vi "Autonomous Independent.vi"() -> ()   [LabVIEW 2016]
doc: "This VI is called when autonomous begins, and will automatically be terminated when autonomous ends. You can carry out timed or sensor driven robot movement independently without needing to return to the caller."
uses:
  <vilib>/Rock Robotics/Network Tables/NT Read Number.vi
  1_25_17/Action_type_def.ctl
  <vilib>/Rock Robotics/WPI/Solenoid/WPI_SolenoidValue.ctl
panel:
  in  "Value":T1=enum."Forward"
  out "Defense Type":dbl=3.0
  in  "Auton_Modes":T3(array[cluster])=[{"Actions"=[{"Action"=enum."Drive", "Effort"=0.55, "Duration"=3.5}, {"Action"=enum."Nothing", "Effort"=0.0, "Duration"=0.0}]}, {"Actions"=[{"Action"=enum."Art Down", "Effort"=0.0, "Duration"=1.0}, {"Action"=enum."Drive", "Effort"=0.75, "Duration"=5.0}, {"Action"=enum."Art Up", "Effort"=0.0, "Duration"=1.0}]}, {"Actions"=[{"Action"=enum."Drive", "Effort"=1.0, "Duration"=3.0}, {"Action"=enum."Art Down", "Effort"=0.0, "Duration"=1.0}, {"Action"=enum."Drive", "Effort"=0.75, "Duration"=3.5}, {"Action"=enum."Art Up", "Effort"=0.0, "Duration"=1.0}]}, {"Actions"=[{"Action"=enum."Art Down", "Effort"=0.0, "Duration"=0.5}, {"Action"=enum."Drive", "Effort"=0.8, "Duration"=5.28}, {"Action"=enum."Art Up", "Effort"=0.0, "Duration"=1.0}, {"Action"=enum."Turn", "Effort"=-0.8, "Duration"=1.8}, {"Action"=enum."Nothing", "Effort"=0.0, "Duration"=0.1}, {"Action"=enum."Drive", "Effort"=0.8, "Duration"=1.75}, {"Action"=enum."Art Down", "Effort"=0.0, "Duration"=0.5}, {"Action"=enum."climb", "Effort"=0.0, "Duration"=4.0}]}, {"Actions"=[{"Action"=enum."Shift", "Effort"=0.0, "Duration"=0.0}, {"Action"=enum."Drive", "Effort"=1.0, "Duration"=0.1}, {"Action"=enum."Nothing", "Effort"=0.0, "Duration"=0.1}, {"Action"=enum."Drive", "Effort"=1.0, "Duration"=3.0}]}, {"Actions"=[{"Action"=enum."Shift", "Effort"=0.0, "Duration"=0.0}, {"Action"=enum."Drive", "Effort"=1.0, "Duration"=0.1}, {"Action"=enum."Nothing", "Effort"=0.0, "Duration"=0.1}, {"Action"=enum."Drive", "Effort"=1.0, "Duration"=3.0}]}, {"Actions"=[{"Action"=enum."Drive", "Effort"=0.55, "Duration"=4.0}, {"Action"=enum."Art Down", "Effort"=0.0, "Duration"=1.0}, {"Action"=enum."Drive", "Effort"=-0.5, "Duration"=0.6}, {"Action"=enum."Drive", "Effort"=0.75, "Duration"=1.0}, {"Action"=enum."Art Up", "Effort"=0.0, "Duration"=1.0}, {"Action"=enum."Drive", "Effort"=0.75, "Duration"=3.0}]}, {"Actions"=[{"Action"=enum."Art Down", "Effort"=0.0, "Duration"=0.5}, {"Action"=enum."Drive", "Effort"=0.55, "Duration"=4.25}, {"Action"=enum."Art Up", "Effort"=0.0, "Duration"=0.0}, {"Action"=enum."Nothing", "Effort"=0.0, "Duration"=0.3}, {"Action"=enum."Drive", "Effort"=0.9, "Duration"=2.0}]}, {"Actions"=[{"Action"=enum."Nothing", "Effort"=0.0, "Duration"=0.0}]}]
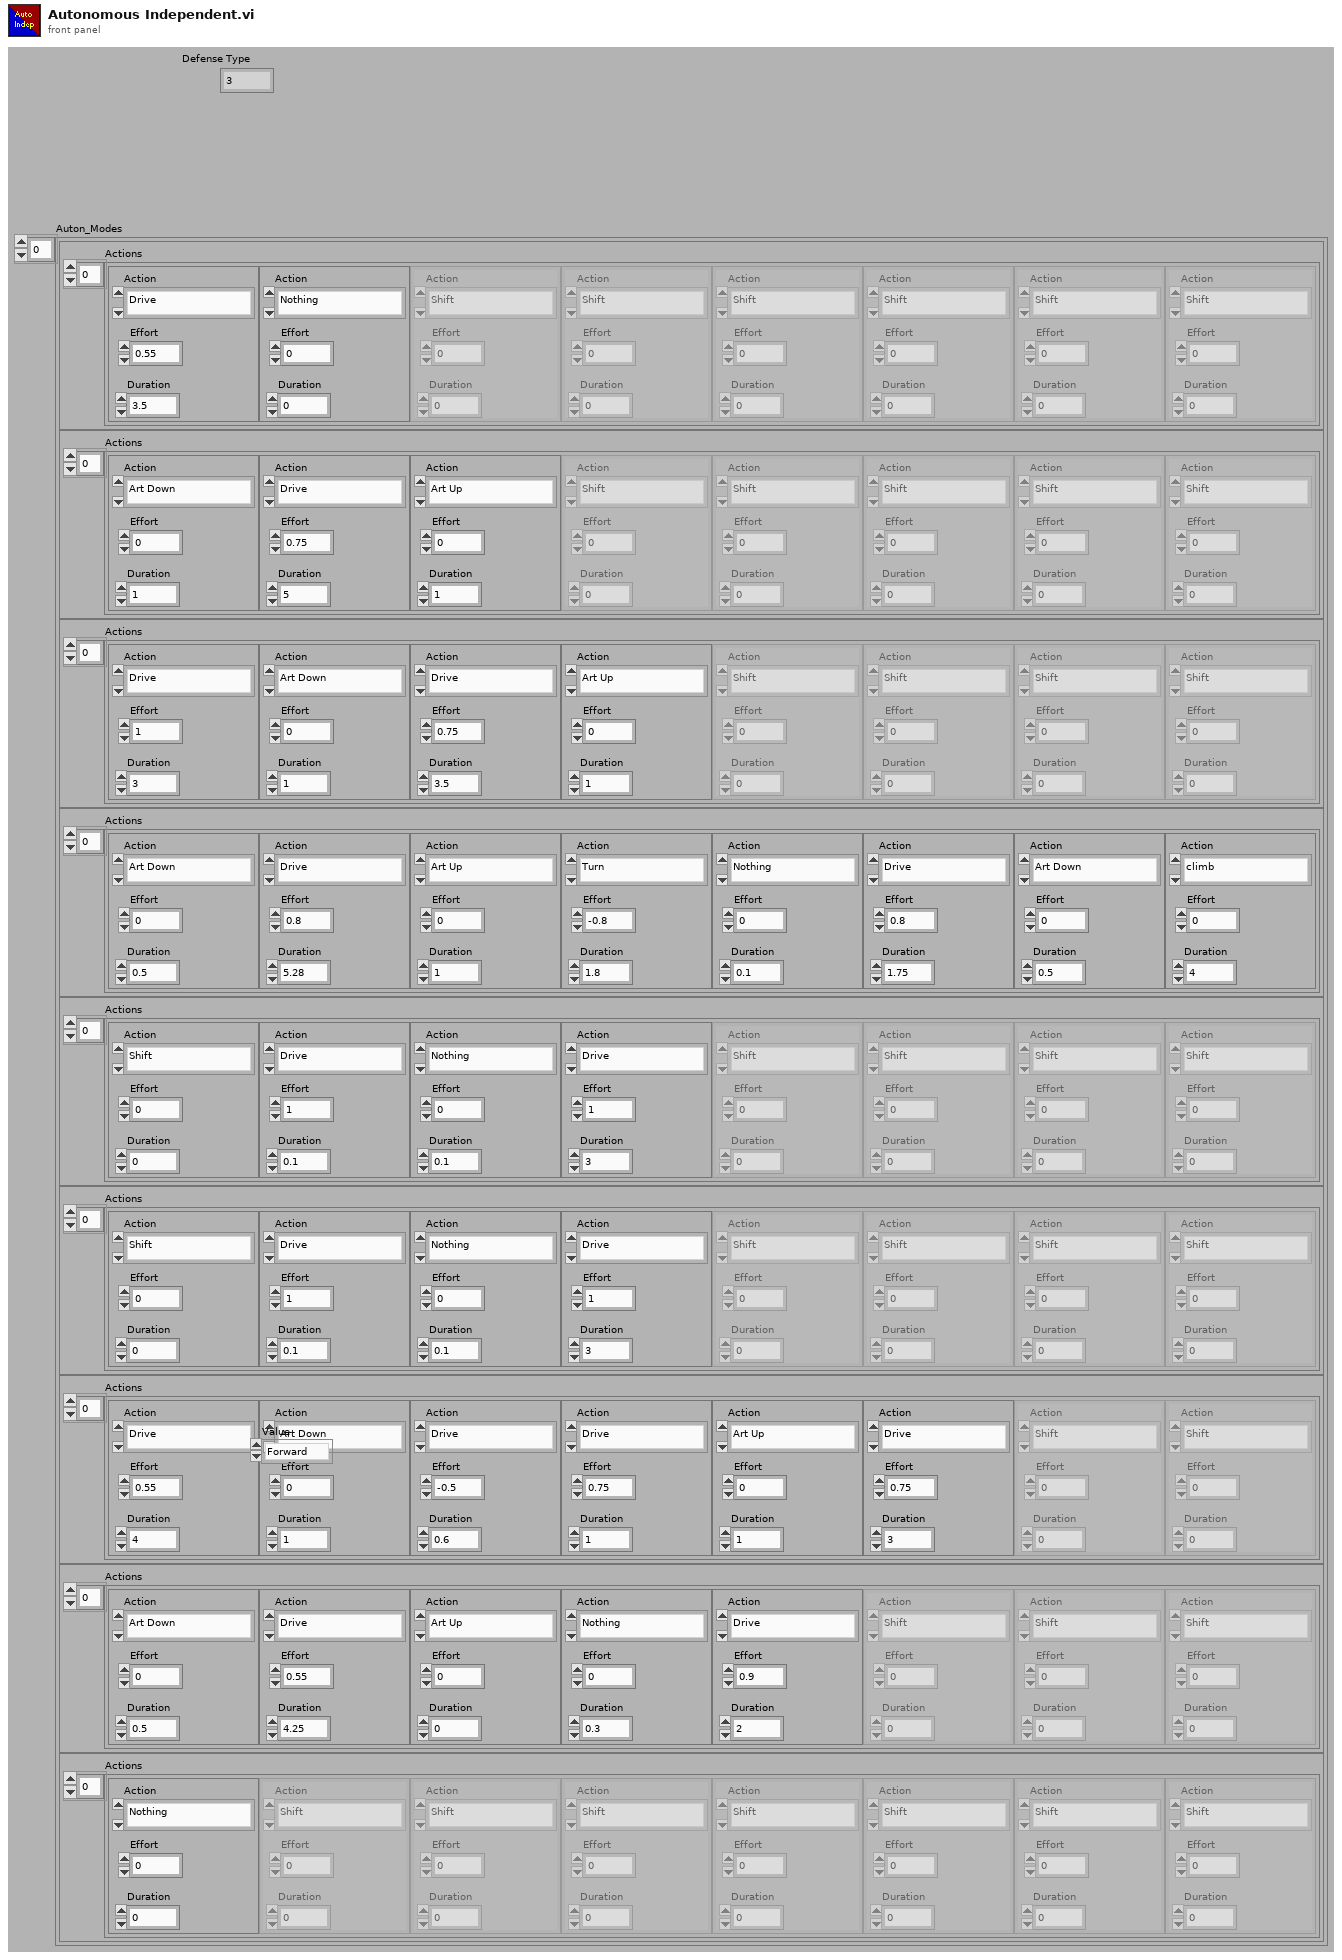
[diagram p1: front panel]
types:
  T1 = typedef "WPI_SolenoidValue.ctl" = enum16{"Off", "On", "Forward", "Reverse"}
  T2 = typedef "Action_type_def.ctl" = enum16{"Shift", "Shoot", "Move Articulates", "Nothing", "Drive", "Turn", "climb", "Art Up", "Art Down", "Test"}
  T3 = cluster{"Actions":cluster{"Action":T2, "Effort":dbl, "Duration":dbl}[]}[]
  T4 = cluster{"Actions":cluster{"Action":T2, "Effort":dbl, "Duration":dbl}[]}
  T5 = cluster{"Action":T2, "Effort":dbl, "Duration":dbl}[]
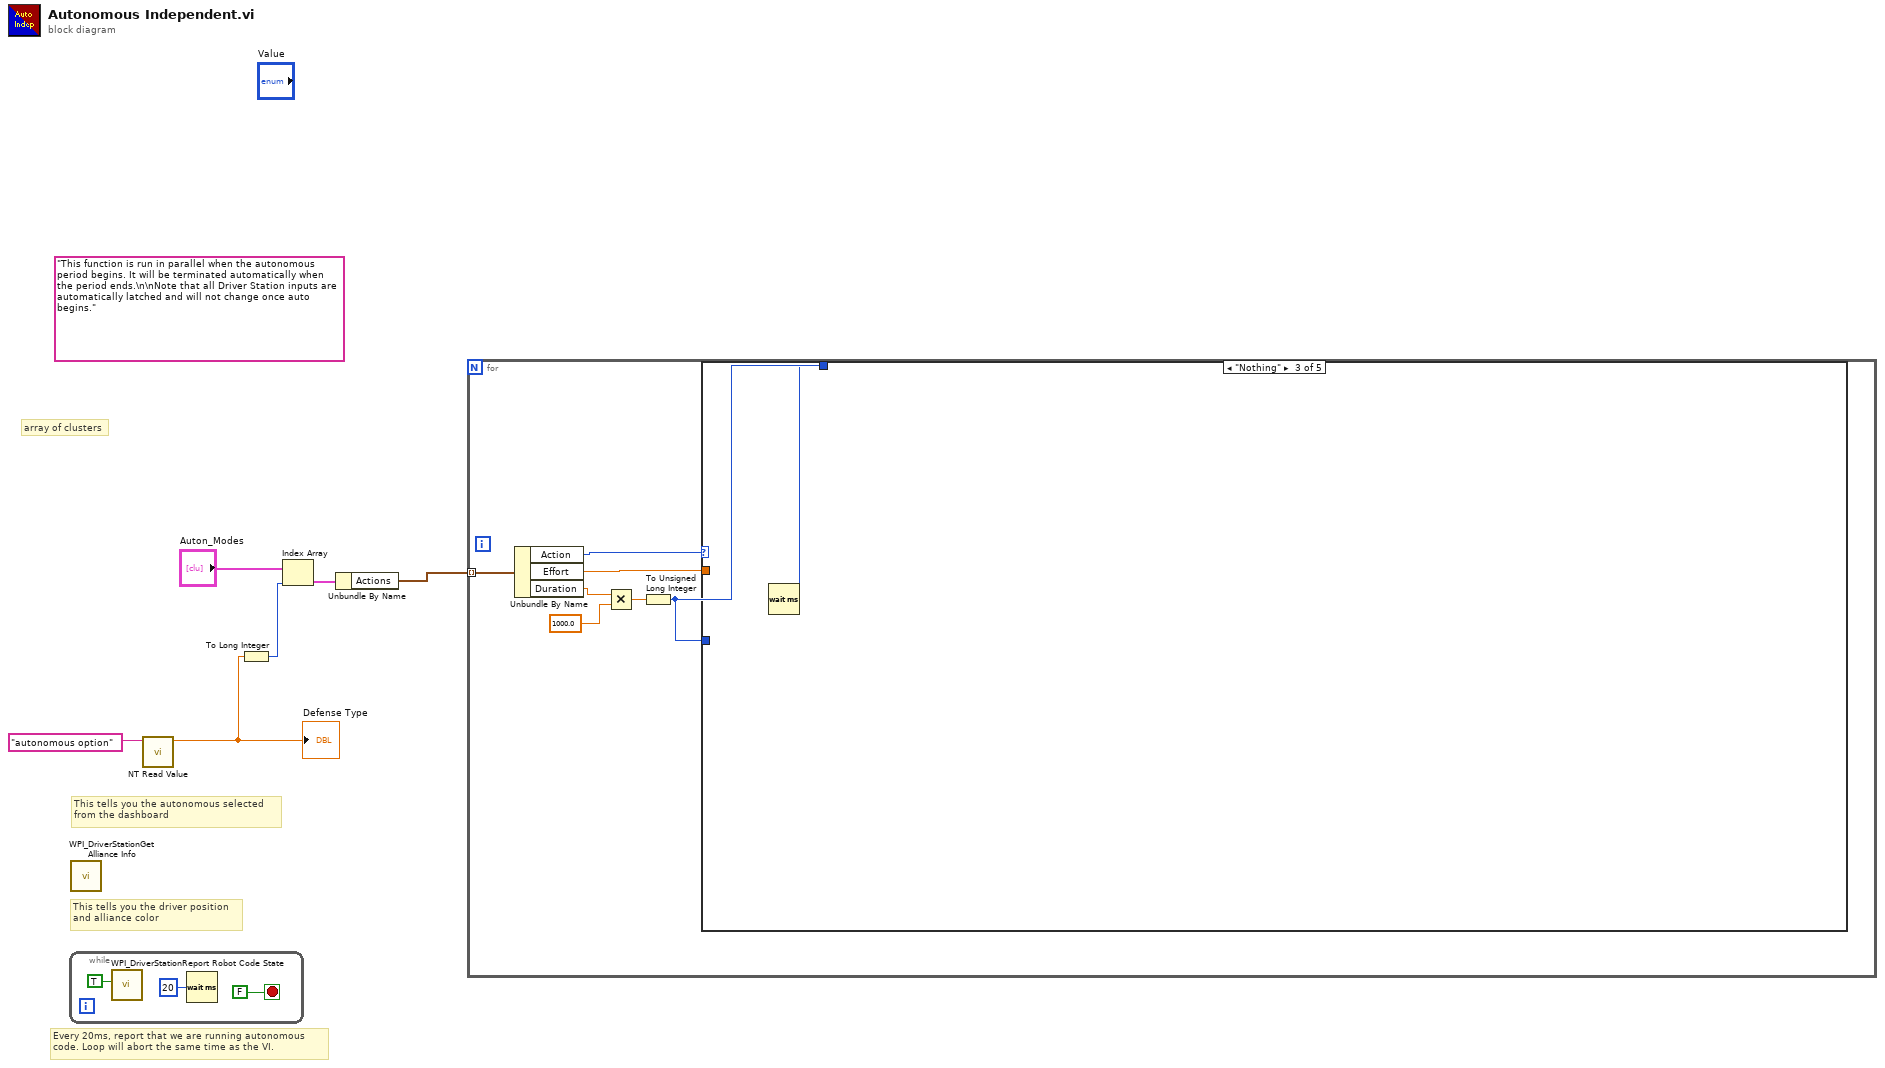
[diagram p0: block diagram]
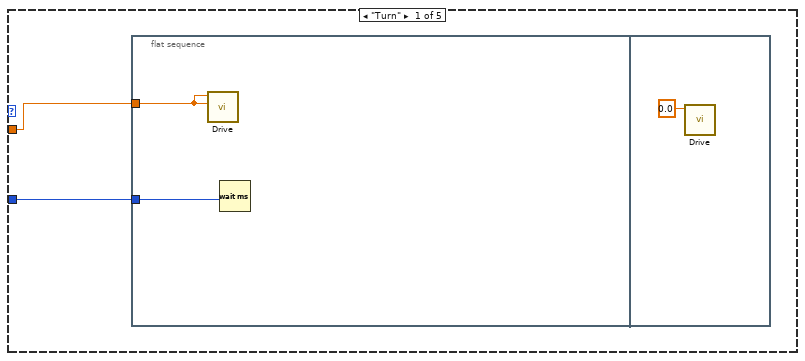
[diagram p2: hidden frame]
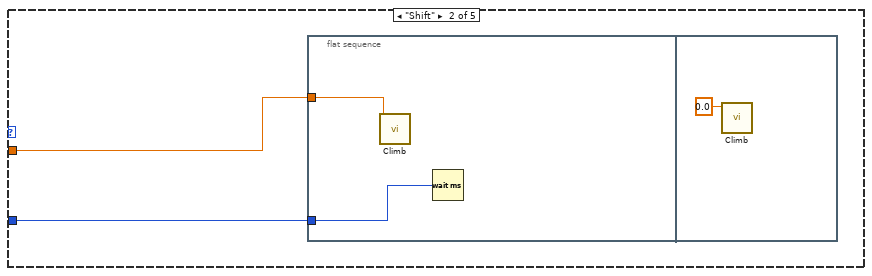
[diagram p3: hidden frame]
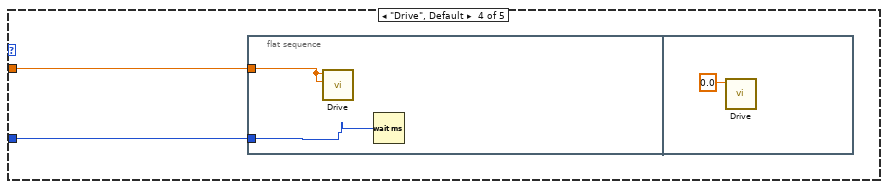
[diagram p4: hidden frame]
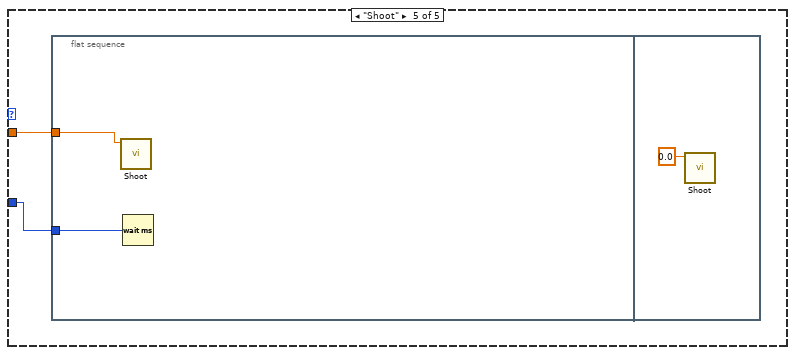
[diagram p5: hidden frame]
diagram:
  (unwired) "This function is run in parallel when the autonomous period begins. It will be terminated automatically when the period ends.\n\nNote that all Driver Station inputs are automatically latched and will not change once auto begins."
  # "This tells you the autonomous selected\nfrom the dashboard"
  # "array of clusters"
  # "Every 20ms, report that we are running autonomous\ncode. Loop will abort the same time as the VI."
  # "This tells you the driver position\nand alliance color"
  n1 = while {
    stop <- FALSE stop-if-true
    n2 = call <vilib>:"WPI_DriverStationReport Robot Code State.vi"("Autonomous"=TRUE) -> ()  [unwired: 10 in, 1 out]
    n3 = Wait (ms)(milliseconds to wait=u32 20) -> ()  [unwired: 1 out]
  }
  n4 = call <vilib>:"WPI_DriverStationGet Alliance Info.vi"() -> ()  [unwired: 12 out]
  n5 = call-poly <vilib>:"NT Read Value.vi"("Name"="autonomous option") -> ("Numeric"=w1:dbl)  [unwired: 9 in, 1 out]
  "Defense Type" <- w1
  n6 = To Long Integer(number=w1) -> (32bit integer=w3:i32)
  n7 = Index Array(array="Auton_Modes", index=w3) -> (element=w5:T4)
  n8 = Unbundle By Name(w5) -> ("Actions"=w6:T5)
  n9 = for {
    tunnel: w6 -> [w16] mode=indexing
    n10 = Unbundle By Name(w16) -> ("Action"=w15:T2, "Effort"=w14:dbl, "Duration"=w13:dbl)
    n11 = Multiply(x=w13, y=1000.0) -> (x*y=w11:dbl)
    n12 = To Unsigned Long Integer(number=w11) -> (unsigned 32bit integer=w10:u32)
    n13 = case shown="\"Nothing\"" w15 {
      tunnel: w14 -> [w18 w23 _ w29 w34]
      tunnel: w10 -> [_ _ w27 _ _]
      tunnel: w10 -> [w17 w22 _ w28 w33]
      frame "Turn" {
        n14 = flat-sequence {
          tunnel: w18 -> [w20]
          tunnel: w17 -> [w19]
          frame #0 {
            n15 = call "Drive.vi"("Drive R"=w20, "Drive L"=w20) -> ()  [unwired: 10 in]
            n16 = Wait (ms)(milliseconds to wait=w19) -> ()  [unwired: 1 out]
          }
          frame #1 {
            n17 = call "Drive.vi"("Drive L"=0.0) -> ()  [unwired: 11 in]
          }
        }
      }
      frame "Shift" {
        n18 = flat-sequence {
          tunnel: w23 -> [w25]
          tunnel: w22 -> [w24]
          frame #0 {
            n19 = call "Climb.vi"("Effort"=w25) -> ()  [unwired: 11 in]
            n20 = Wait (ms)(milliseconds to wait=w24) -> ()  [unwired: 1 out]
          }
          frame #1 {
            n21 = call "Climb.vi"("Effort"=0.0) -> ()  [unwired: 11 in]
          }
        }
      }
      frame "Nothing" {
        n22 = Wait (ms)(milliseconds to wait=w27) -> ()  [unwired: 1 out]
      }
      frame "Drive", Default {
        n23 = flat-sequence {
          tunnel: w29 -> [w31]
          tunnel: w28 -> [w30]
          frame #0 {
            n24 = call "Drive.vi"("Drive R"=w31, "Drive L"=w31) -> ()  [unwired: 10 in]
            n25 = Wait (ms)(milliseconds to wait=w30) -> ()  [unwired: 1 out]
          }
          frame #1 {
            n26 = call "Drive.vi"("Drive L"=0.0) -> ()  [unwired: 11 in]
          }
        }
      }
      frame "Shoot" {
        n27 = flat-sequence {
          tunnel: w34 -> [w36]
          tunnel: w33 -> [w35]
          frame #0 {
            n28 = call "Shoot.vi"("Effort"=w36) -> ()  [unwired: 11 in]
            n29 = Wait (ms)(milliseconds to wait=w35) -> ()  [unwired: 1 out]
          }
          frame #1 {
            n30 = call "Shoot.vi"("Effort"=0.0) -> ()  [unwired: 11 in]
          }
        }
      }
    }
  }
